vi "lab3_task4.vi"() -> ()   [LabVIEW 2021]
uses:
  <vilib>/express/express analysis/Spectral/Block/exnSpectralBlock spectral measurements PSD poly.vi
  <vilib>/express/express analysis/Spectral/Block/exnSpectralBlock spectral measurements PSD DDT.vi
  <vilib>/express/express analysis/Spectral/XNode/ExpressSpectralMeasurementsBlockNode.xnode
  <vilib>/Analysis/NI_AALPro.lvlib
panel:
  out "number samples":dbl
  in  "Duration":dbl=10000.0
  in  "Sampling rate":dbl=10000.0
  in  "stop":bool
  out "Intensity Chart":dbl[][](graph)
  out "Power spectral density":dynamicdata(graph)
  in  "# bins":i32
  out "Histogram Graph":T1(graph)
  out "rms":dbl
  out "peak to peak":dbl
  out "mean":dbl
  out "data":dynamicdata(graph)
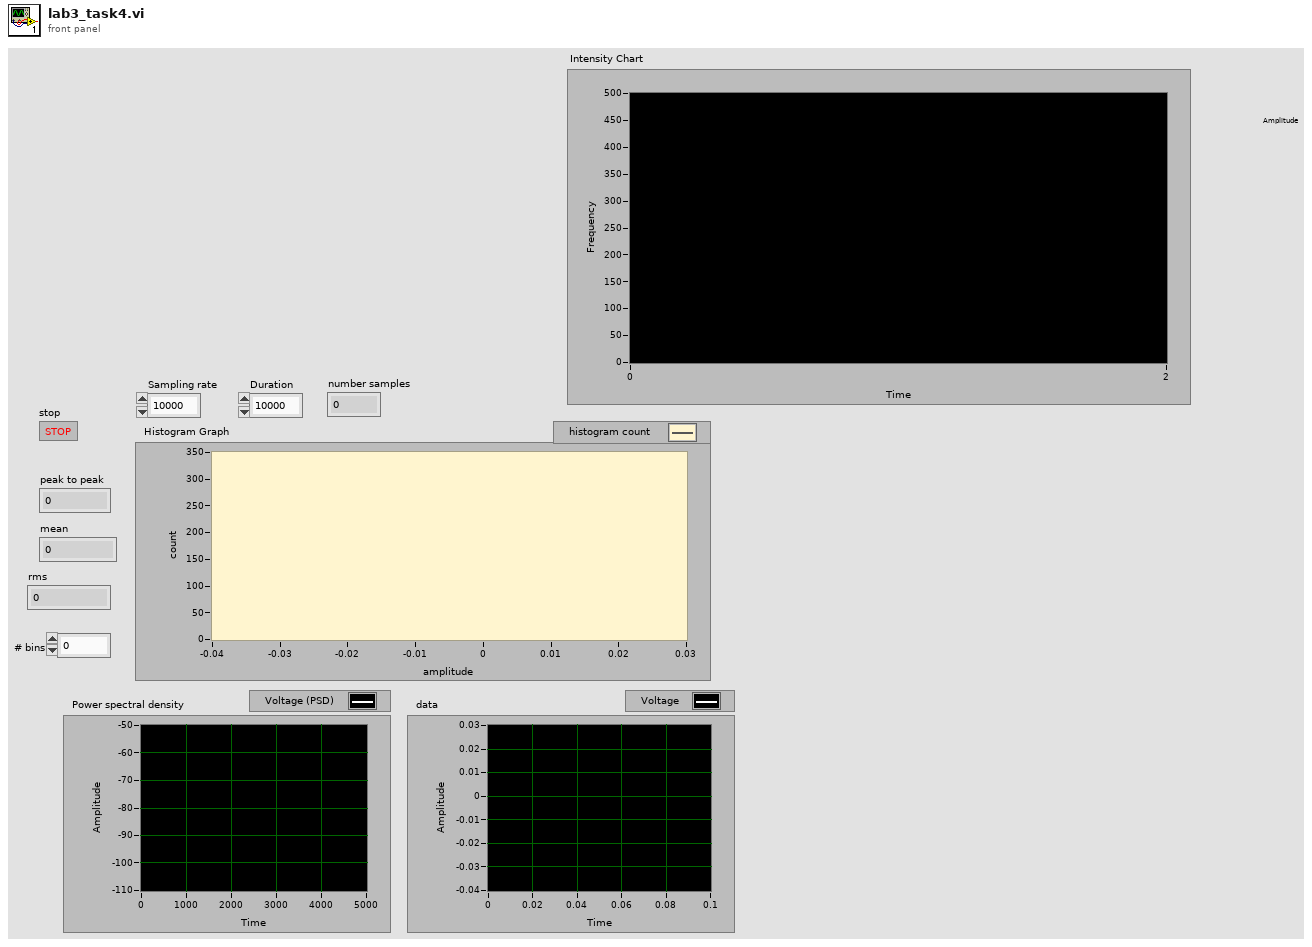
[diagram p1: front panel]
types:
  T1 = cluster{"X Values":dbl[], "Histogram: h(x)":i32[]}
  T2 = cluster{"averaging mode":u16, "weighting mode":u16, "number of averages":u32}
  T3 = cluster{"dB On (F)":bool, "unwrap phase (F)":bool, "convert to degree (F)":bool}
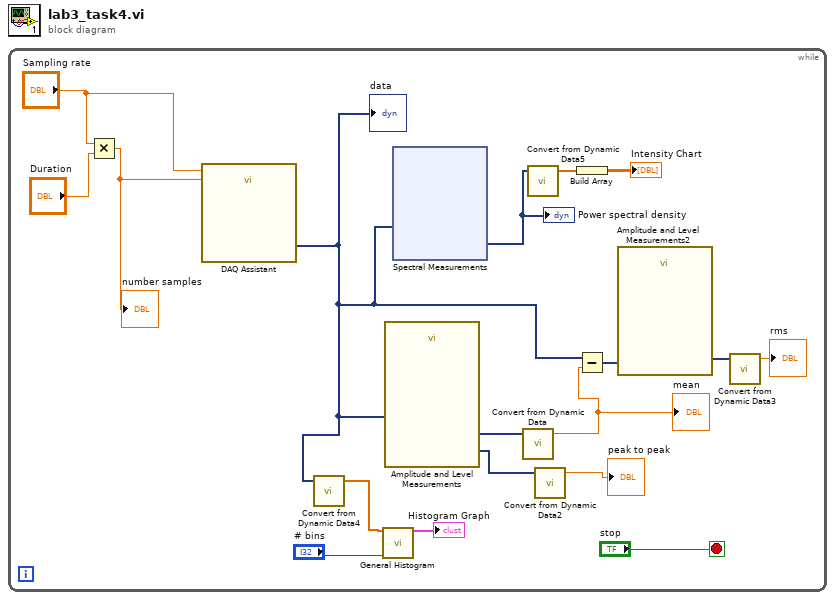
[diagram p0: block diagram]
diagram:
  n1 = while {
    stop <- "stop" stop-if-true
    n2 = Multiply(x="Sampling rate", y="Duration") -> (x*y=w1:dbl)
    "number samples" <- w1
    n3 = call "DAQ Assistant"("rate"="Sampling rate", "number of samples"=w1) -> ("data"=w8:dynamicdata)  [unwired: 15 in, 2 out]
    "data" <- w8
    n4 = call "Convert from Dynamic Data4"("Dynamic Data Type"=w8) -> ("Array"=w9:dbl[])  [unwired: 3 in]
    n5 = call <vilib>:"General Histogram.vi"("X"=w9, "# bins"="# bins") -> ("Histogram Graph"=→"Histogram Graph":T1)  [unwired: 9 in, 4 out]
    n6 = call "Amplitude and Level Measurements"("Signals"=w8) -> ("Mean (DC)"=w18:dynamicdata, "Peak to Peak"=w17:dynamicdata)  [unwired: 12 in, 1 out]
    n7 = xnode "Spectral Measurements"("Signals"=w8) -> ("PSD"=w7:dynamicdata)  [unwired: 1 in, 1 out]
    "Power spectral density" <- w7
    n8 = call "Convert from Dynamic Data"("Dynamic Data Type"=w18) -> ("Scalar"=w15:dbl)  [unwired: 3 in]
    "mean" <- w15
    n9 = call "Convert from Dynamic Data5"("Dynamic Data Type"=w7) -> ("Array"=w6:dbl[])  [unwired: 3 in]
    n10 = call "Convert from Dynamic Data2"("Dynamic Data Type"=w17) -> ("Scalar"=→"peak to peak":dbl)  [unwired: 3 in]
    n11 = Build Array(w6) -> (→"Intensity Chart":dbl[][])
    n12 = Subtract(x=w8, y=w15) -> (x-y=w14:dynamicdata)
    n13 = call "Amplitude and Level Measurements2"("Signals"=w14) -> ("RMS"=w13:dynamicdata)  [unwired: 13 in, 1 out]
    n14 = call "Convert from Dynamic Data3"("Dynamic Data Type"=w13) -> ("Scalar"=→"rms":dbl)  [unwired: 3 in]
  }
